vi "Build Resistor Section from XML.vi"(6 "Channels":refnum<k24>[](array[refnum]), 8 "error in (no error)":errorcluster, 9 "Card Position":T1 {"Slot #" max=15}, 10 "Name":string, 11 "Node Ptr":u64) -> (0 "error out":errorcluster)   [LabVIEW 2014, in "SLSC configuration System Explorer.lvlib"]
uses:
  SLSC configuration System Explorer.lvlib
  Type Defs/Card Position.ctl
  Shared/SPI Utility/Slot #.ctl
  C:/Files/Custom VeriStand Development/DET-SPI-Tool/XML Deserializer/SLSC Deserializer/SLSC Deserializer/bin/Release/SLSC Deserializer.dll
  XML Deserializer/SLSC Deserializer/SLSC Deserializer/bin/Release/SLSC Deserializer.dll
  <vilib>/NI Veristand/Custom Device API/Custom Device Channel.ctl
  <vilib>/NI Veristand/Custom Device API/Custom Device Channel Type.ctl
  Shared/Constants.vi
  <vilib>/NI Veristand/Custom Device API/Set Item Property (U16).vi
  <vilib>/NI Veristand/Custom Device API/Custom Device API.lvlib
  Shared/SLSC configuration Shared.lvlib
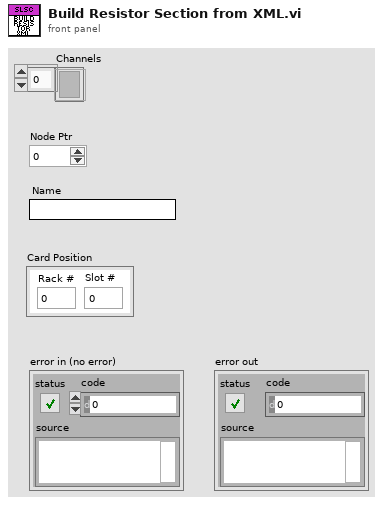
[diagram p1: front panel]
types:
  T1 = typedef "SLSC configuration Shared.lvlib/Card Position.ctl" = cluster{"Rack #":u8, "Slot #":T2}
  T2 = typedef "SLSC configuration Shared.lvlib/Slot #.ctl" = u8
  T3 = typedef "Custom Device API.lvlib/Custom Device Channel Type.ctl" = enum16{"Input", "Output"}
  T4 = typedef "Custom Device API.lvlib/Custom Device Channel.ctl" = cluster{"Type":T3, "Units":string, "Default Value":dbl, "Faultable":bool, "Scalable":bool}
  T5 = typedef "Custom Device API.lvlib/Custom Device Item Ref.ctl" = u64
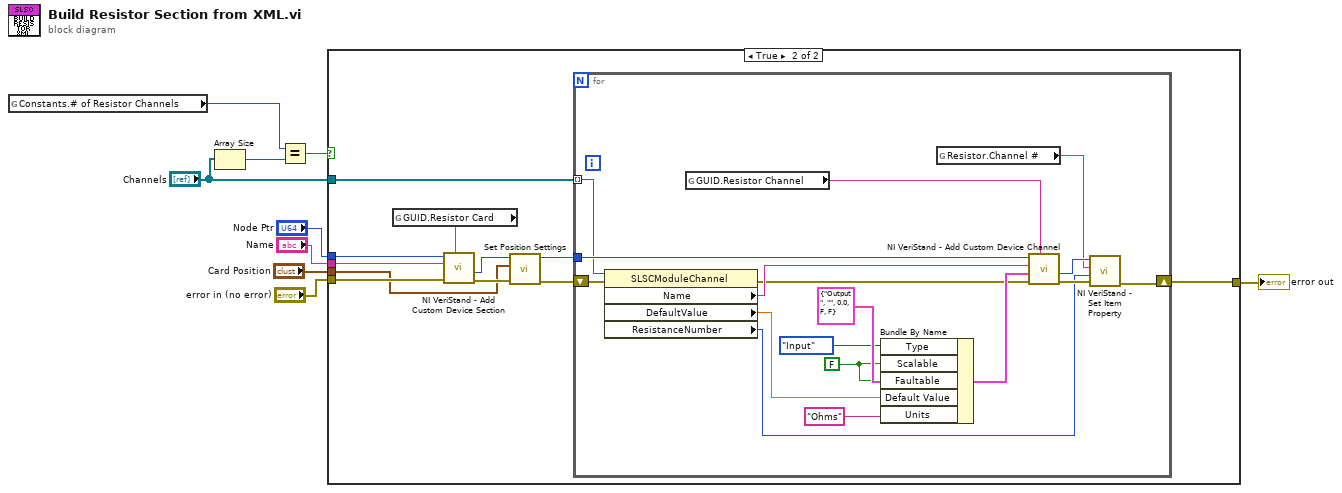
[diagram p0: block diagram]
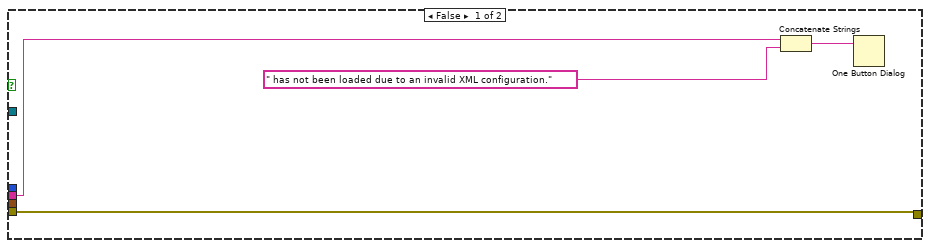
[diagram p2: hidden frame]
diagram:
  n1 = global read "Constants.vi" "Constants.# of Resistor Channels"() -> (w3:u8)
  n2 = Array Size(array="Channels") -> (size(s)=w4:i32)
  n3 = Equal?(x=w3, y=w4) -> (x = y?=w2:bool)
  n4 = case shown="True" w2 {
    tunnel: "error in (no error)" -> [w13 w24]
    tunnel: "Node Ptr" -> [_ w23]
    tunnel: "Card Position" -> [_ w20]
    tunnel: [w13 w15] -> w7
    tunnel: "Name" -> [w10 w16]
    tunnel: "Channels" -> [_ w14]
    frame False {
      n5 = Concatenate Strings(w10, " has not been loaded due to an invalid XML configuration." ("string")) -> (w11:string)
      n6 = One Button Dialog(message=w11) -> ()  [unwired: 1 in, 1 out]
    }
    frame True {
      n7 = global read "Constants.vi" "GUID.Resistor Card"() -> (w22:string)
      n8 = call <vilib>:"NI VeriStand - Add Custom Device Section.vi"("GUID (Default Section)"=w22, "error in (no error)"=w24, "Section Name"=w16, "Parent Ref in"=w23) -> ("error out"=w21:errorcluster, "Section Ptr"=w19:T5)  [unwired: 4 in, 2 out]
      n9 = call "Set Position Settings.vi"("error in (no error)"=w21, "Card Position"=w20, "Item Ref in"=w19) -> ("error out"=w18:errorcluster, "Item Ref out"=w17:T5)  [unwired: 7 in]
      n10 = for {
        shift-right: [w32] -> w15
        shift-left: w18 -> [w30]
        tunnel: w17 -> [w35]
        tunnel: w14 -> [w29] mode=indexing
        w38 = FALSE ("Scalable")
        n11 = property class="SLSCModuleChannel"(reference=w29, error in=w30) -> (error out=w27:errorcluster, "Name"=w28:string, "DefaultValue"=w26:dbl, "ResistanceNumber"=w25:u8)  [unwired: 1 out]
        n12 = global read "Constants.vi" "GUID.Resistor Channel"() -> (w37:string)
        n13 = Bundle By Name(cluster=T4 {"Type"=enum."Output", "Units"="", "Default Value"=0.0, "Faultable"=FALSE, "Scalable"=FALSE} ("Channel"), "Type"=Custom_Device_Channel_Type."Input", "Scalable"=w38, "Faultable"=w38, "Default Value"=w26, "Units"="Ohms") -> (w40:T4)
        n14 = global read "Constants.vi" "Resistor.Channel #"() -> (w33:string)
        n15 = call <vilib>:"NI VeriStand - Add Custom Device Channel.vi"("GUID (Default Channel)"=w37, "error in (no error)"=w27, "Channel"=w40, "Channel Name"=w28, "Parent Ref in"=w35) -> ("error out"=w36:errorcluster, "Channel Ref"=w34:T5)  [unwired: 3 in, 2 out]
        n16 = call-poly <vilib>:"NI VeriStand - Set Item Property.vi"("error in (no error)"=w36, "Value"=w25, "Property Name"=w33, "Item Ref in"=w34) -> ("error out"=w32:errorcluster)  [unwired: 5 in, 2 out]
      }
    }
  }
  "error out" <- w7
